vi "MeasureChannel.vi"(8 "error in (no error)":errorcluster, 9 "MainMsg":T1, 10 "MainQueue in":refnum<queue>, 11 "Channel In":refnum<k21>) -> (0 "error out":errorcluster, 2 "MainQueue out":refnum<queue>)   [LabVIEW 2017]
uses:
  MainMsg.ctl
  CTRLS/MainCluster.ctl
  <vilib>/DAQmx/read.llb/DAQmx Read (Analog DBL 1Chan 1Samp).vi
  <vilib>/DAQmx/miscellaneous.llb/DAQmx Fill In Error Info.vi
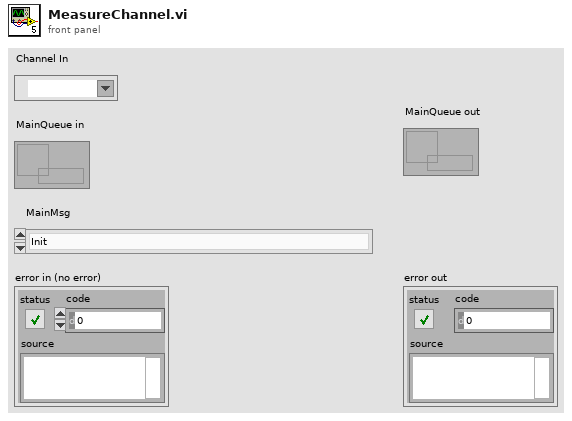
[diagram p1: front panel]
types:
  T1 = typedef "MainMsg.ctl" = enum16{"Init", "Halt", "MonitorState", "SaveState", "Filename", "AirFlow", "WaterFlow", "AirPress", "WaterPress", "WaterTemp", "NozzleForce", "SaveAll", "Error", "Supervisor"}
  T2 = typedef "MainCluster.ctl" = cluster{"MainMsg":T1, "MainNum":dbl, "MainStr":string}
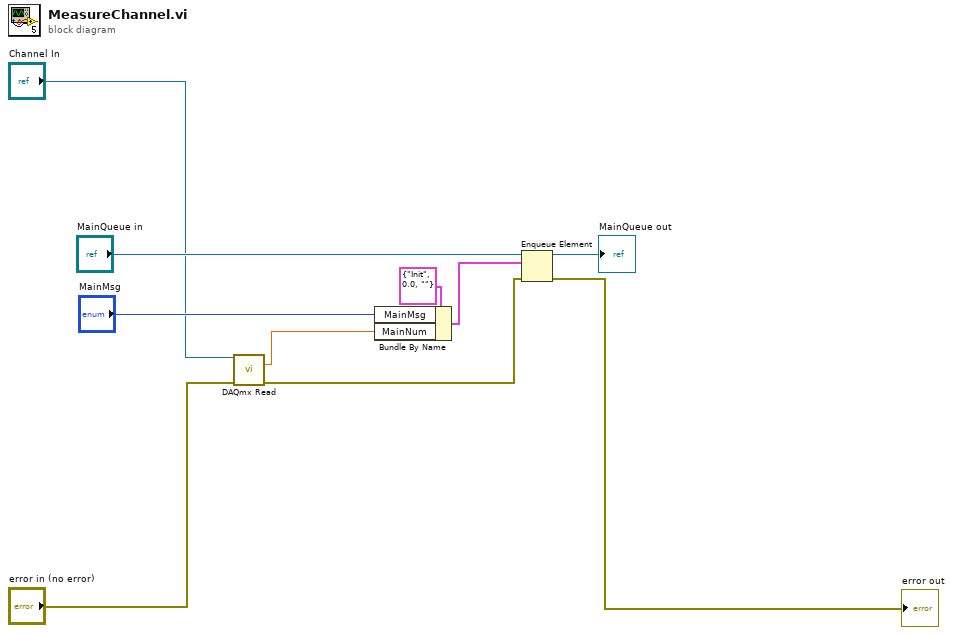
[diagram p0: block diagram]
diagram:
  n1 = call-poly <vilib>:"DAQmx Read.vi"("task/channels in"="Channel In", "error in"="error in (no error)") -> ("data"=w8:dbl, "error out"=w5:errorcluster)  [unwired: 11 in, 1 out]
  n2 = Bundle By Name(cluster=T2 {"MainMsg"=enum."Init", "MainNum"=0.0, "MainStr"=""} ("element"), "MainMsg"="MainMsg", "MainNum"=w8) -> (w9:T2)
  n3 = Enqueue Element(queue="MainQueue in", element=w9, error in (no error)=w5) -> (queue out=→"MainQueue out":refnum<queue>, error out=→"error out":errorcluster)  [unwired: 1 in, 1 out]
